vi "Write Error.vi"(10 "Error":string, 11 "Result in":refnum<class "Result.lvclass">) -> (3 "Result out":refnum<class "Result.lvclass">)   [LabVIEW 2018, in "InfluxDB Client.lvlib" / "Result.lvclass"]
uses:
  Result.lvclass
  Result.lvclass/Result.ctl
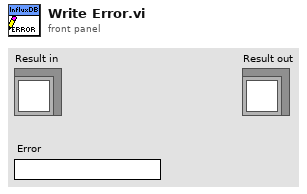
[diagram p1: front panel]
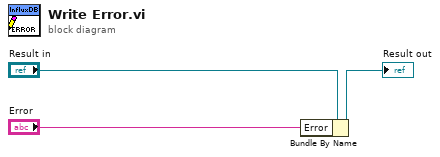
[diagram p0: block diagram]
diagram:
  n1 = Bundle By Name(cluster="Result in", "Error"="Error") -> (→"Result out":refnum<class "Result.lvclass">)
